vi "Get Image from VI Ref.vi"(8 "error in (no error)":errorcluster, 11 "VI Reference Control in":refnum<class "VI Reference Control.lvclass">) -> (0 "error out":errorcluster, 2 "new picture":picture, 3 "VI Reference Control out":refnum<class "VI Reference Control.lvclass">)   [LabVIEW 2016, in "VI Reference Control.lvclass"]
uses:
  VI Reference Control.lvclass
  VI Reference Control.lvclass/VI Reference Control.ctl
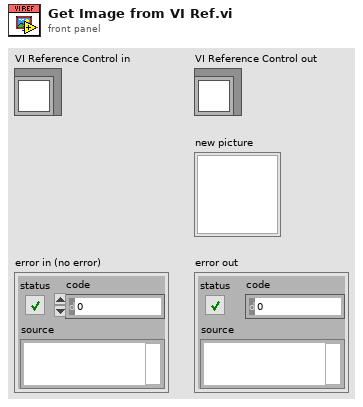
[diagram p1: front panel]
types:
  T1 = typedef "imagedata.ctl" = cluster{"image type":i32, "image depth":i32, "image":u8[], "mask":u8[], "colors":u32[], "Rectangle":cluster{"left":i16, "top":i16, "right":i16, "bottom":i16}}
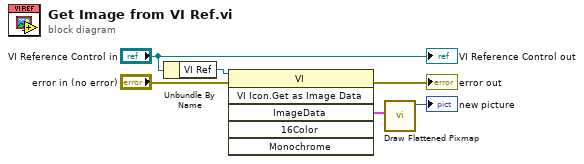
[diagram p0: block diagram]
diagram:
  n1 = Unbundle By Name("VI Reference Control in") -> ("VI Ref"=w1:refnum<vi>)
  n2 = invoke class="VI" method="VI Icon.Get as Image Data"(reference=w1, error in="error in (no error)") -> (error out=→"error out":errorcluster, "ImageData"=w3:T1)  [unwired: 4 in, 4 out]
  n3 = call <vilib>:"Draw Flattened Pixmap.vi"("image data"=w3) -> ("new picture"=→"new picture":picture)  [unwired: 8 in]
  "VI Reference Control out" <- "VI Reference Control in"
